vi "InitializeLowRateCountTag.vi"(10 "Group":string, 11 "Device":string) -> (3 "LowRateCountTag":T1)   [LabVIEW 2017, in "DataAccumulator.lvlib"]
uses:
  <vilib>/addons/InsightCM/Devices/Shared/Common/DataAccumulator/DataAccumulator.lvlib
  <vilib>/addons/InsightCM/Devices/Shared/Common/DeviceHealth/controls/deviceHealthTag.ctl
  <vilib>/addons/InsightCM/Devices/Shared/Common/DeviceHealth/controls/SystemHealthTagEnum.ctl
  <vilib>/addons/InsightCM/MessageBus/Base/controls/Tag.ctl
  <vilib>/addons/InsightCM/MessageBus/Base/controls/KeyValuePair.ctl
  <vilib>/addons/InsightCM/Devices/Shared/Common/DeviceHealth/DeviceHealth.lvlib
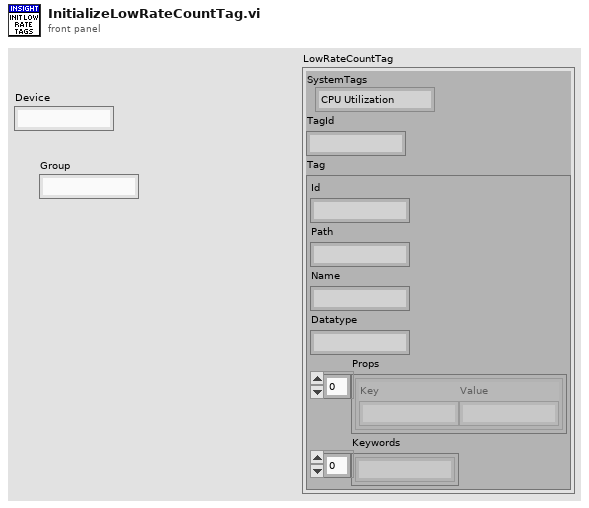
[diagram p1: front panel]
types:
  T1 = typedef "DeviceHealth.lvlib/deviceHealthTag.ctl" = cluster{"SystemTags":T2, "TagId":string, "Tag":T3}
  T2 = typedef "DeviceHealth.lvlib/SystemHealthTagEnum.ctl" = enum16{"CPU Utilization", "Memory Utilization", "Disk Utilization", "Total Physical Memory", "Primary Disk Free", "Chassis Temperature", "LowRateCount"}
  T3 = typedef "Tag.ctl" = cluster{"Id":string, "Path":string, "Name":string, "Datatype":string, "Props":T4[], "Keywords":string[]}
  T4 = typedef "KeyValuePair.ctl" = cluster{"Key":string, "Value":string}
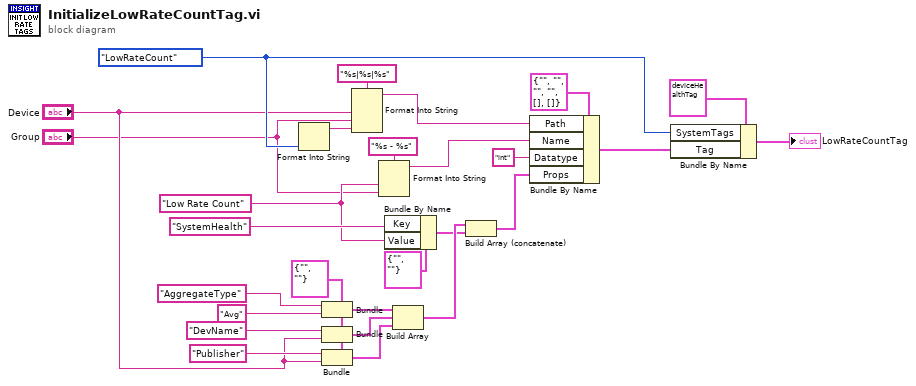
[diagram p0: block diagram]
diagram:
  w4 = "Low Rate Count" ("SearchKey.Key")
  w18 = SystemHealthTagEnum."LowRateCount" ("SystemTags")
  w27 = T4 {"Key"="", "Value"=""}
  n1 = Format Into String(w18) -> (resulting string=w5:string)  [unwired: 3 in, 1 out]
  n2 = Bundle(cluster=w27, "Key"="AggregateType" ("SearchKey.Key"), "Value"="Avg" ("SearchKey.Key")) -> (w26:T4)
  n3 = Bundle(cluster=w27, "Key"="DevName" ("SearchKey.Key"), "Value"="Device") -> (w25:T4)
  n4 = Bundle(cluster=w27, "Key"="Publisher" ("SearchKey.Key"), "Value"="Device") -> (w24:T4)
  n5 = Format Into String(format string="%s|%s|%s", "Device", "Group", w5) -> (resulting string=w9:string)  [unwired: 2 in, 1 out]
  n6 = Format Into String(format string="%s - %s", w4, "Group") -> (resulting string=w1:string)  [unwired: 2 in, 1 out]
  n7 = Bundle By Name(cluster=T4 {"Key"="", "Value"=""}, "Key"="SystemHealth" ("SearchKey.Key"), "Value"=w4) -> (w13:T4)
  n8 = Build Array(w26, w25, w24) -> (w19:T4[])
  n9 = Build Array (concatenate)(w19, w13) -> (w12:T4[])
  n10 = Bundle By Name(cluster=T3 {"Id"="", "Path"="", "Name"="", "Datatype"="", "Props"=[], "Keywords"=[]} ("Tag"), "Path"=w9, "Name"=w1, "Datatype"="int", "Props"=w12) -> (w7:T3)
  n11 = Bundle By Name(cluster=T1 {"SystemTags"=enum."CPU Utilization", "TagId"="", "Tag"={"Id"="", "Path"="", "Name"="", "Datatype"="", "Props"=[], "Keywords"=[]}} ("DeviceHealthTag"), "SystemTags"=w18, "Tag"=w7) -> (→"LowRateCountTag":T1)
